vi "CheckIfNumberIsEven.vi"(11 "x":dbl) -> (3 "even?":bool)   [LabVIEW 2013]
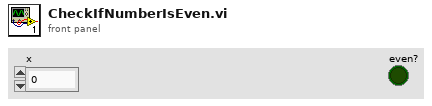
[diagram p1: front panel]
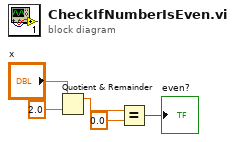
[diagram p0: block diagram]
diagram:
  n1 = Quotient & Remainder(x="x", y=2.0) -> (x-y*floor(x/y)=w3:dbl)  [unwired: 1 out]
  n2 = Equal?(x=w3, y=0.0) -> (x = y?=→"even?":bool)
